vi "TestAxes.vi"(8 "error in (no error)":errorcluster) -> (0 "error out":errorcluster)   [LabVIEW 2009]
uses:
  typedefs/Position3d.ctl
  typedefs/AxesTestSettings.ctl
  typedefs/Ultra3000/Fault_Cluster.ctl
  typedefs/Ultra3000/RunStatus_Ring.ctl
  typedefs/Ultra3000/IndexType.ctl
  typedefs/Ultra3000/HostControlModeRing.ctl
  typedefs/AxisSelect_Enum.ctl
  typedefs/Ultra3000/Index_Numeric.ctl
  typedefs/Ultra3000/IndexTermination.ctl
  typedefs/Ultra3000/AdditionalIndexSettings_Cluster.ctl
panel:
  in  "Y Enable toggle":bool
  in  "Z Enable Toggle":bool
  in  "X Enable toggle":bool
  in  "Axis Settings":T1=[{"Velocity"=5.0, "Accel. / Decel."=5.0, "Dwell"=0}, {"Velocity"=5.0, "Accel. / Decel."=5.0, "Dwell"=0}, {"Velocity"=5.0, "Accel. / Decel."=5.0, "Dwell"=0}]
  in  "Index Type (Absolute)":T2=1 items=["Incremental", "Absolute"]
  in  "Home":bool
  in  "Position 2 (mm)":T3
  in  "Position 1 (mm)":T3
  out "Current (X,Y,Z) Position":string
  in  "stop":bool
  in  "cycle":bool caption="(Hold to start)"
  in  "Move to pos2":bool
  in  "Move to pos1":bool
  in  "Clear Faults":bool
  out "Run Status":T4[](array[typedef]) {"Run Status Description" items=["Fault detected"=1, "Disabled and not faulted"=255, "Enabled"=0]}
  in  "Done":bool
  # "X-Axis Settings"
  # "Y-Axis Settings"
  # "Z-Axis Settings"
  # "X-Axis Run Status"
  # "Y-Axis Run Status"
  # "Z-Axis Run Status"
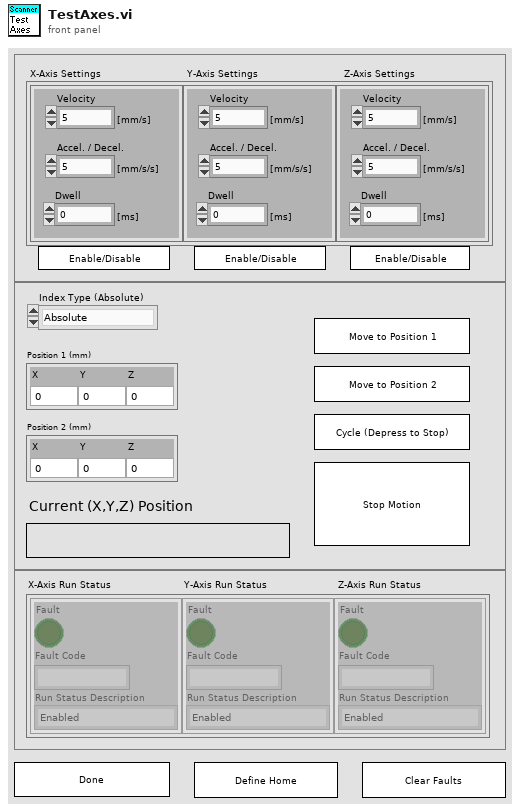
[diagram p1: front panel]
types:
  T1 = typedef "AxesTestSettings.ctl" = cluster{"Velocity":dbl, "Accel. / Decel.":dbl, "Dwell":u16}[]
  T2 = typedef "IndexType.ctl" = i32
  T3 = typedef "Position3d.ctl" = cluster{"X":dbl, "Y":dbl, "Z":dbl}
  T4 = typedef "Fault_Cluster.ctl" = cluster{"Fault":bool, "Fault Code":string, "Run Status Description":T5}
  T5 = typedef "RunStatus_Ring.ctl" = u16
  T6 = typedef "AxisSelect_Enum.ctl" = enum16{"X", "Y", "Z", "Axis Space"}
  T7 = typedef "HostControlModeRing.ctl" = u16
  T8 = typedef "Index_Numeric.ctl" = u8
  T9 = typedef "DriveStatus_Cluster.ctl" = cluster{"In-position":bool, "Zero Speed":bool, "Enabled":bool, "Fault Disable":bool, "Ready":bool, "Start Index":bool, "Overtravel Exceeded":bool, "Up to Speed":bool, "Sequence Complete":bool}
  T10 = enum8{"Enabled", "Disabled", "Disabled and Grayed Out"}
  T11 = typedef "IndexTermination.ctl" = i32
  T12 = typedef "AdditionalIndexSettings_Cluster.ctl" = cluster{"Next Index":u8, "Termination":T11, "Count":u16}
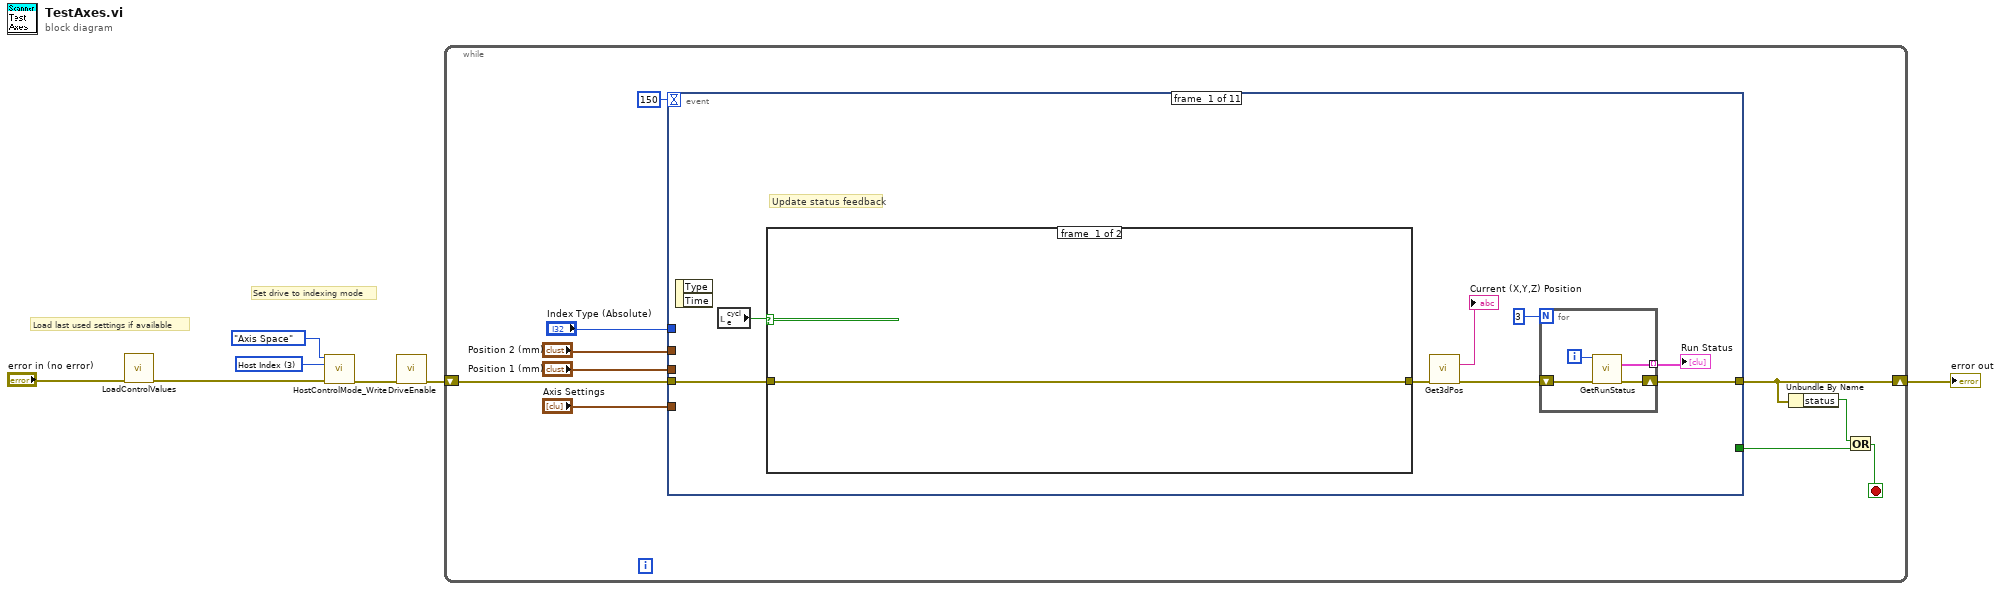
[diagram p0: block diagram]
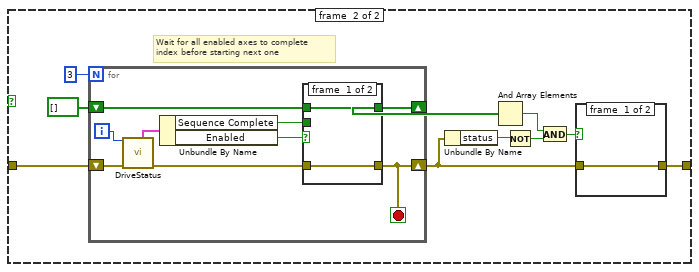
[diagram p2: hidden frame]
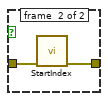
[diagram p3: hidden frame]
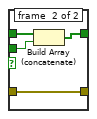
[diagram p4: hidden frame]
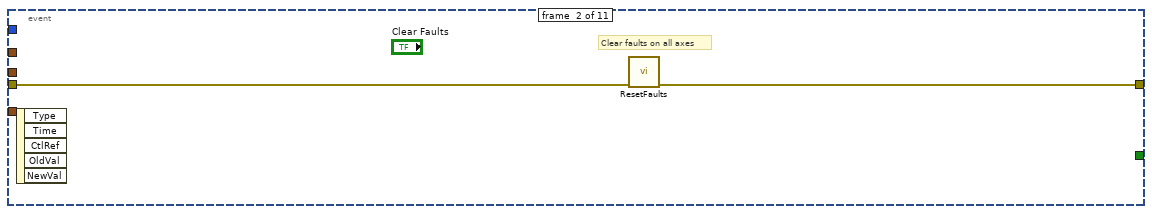
[diagram p5: hidden frame]
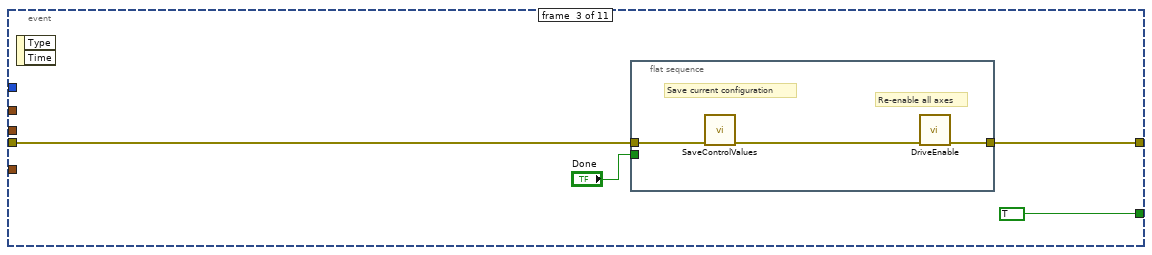
[diagram p6: hidden frame]
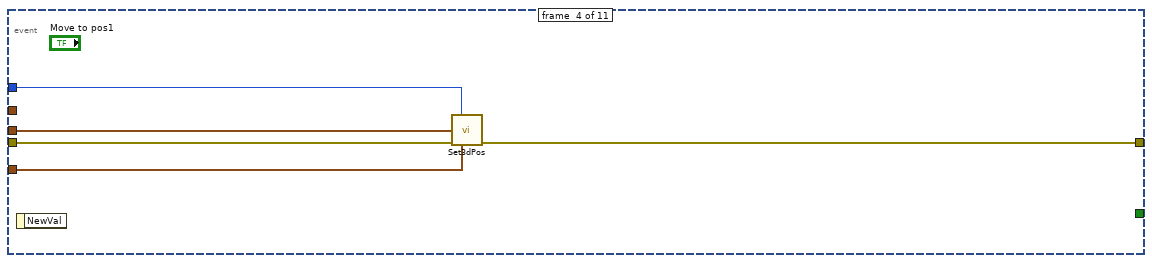
[diagram p7: hidden frame]
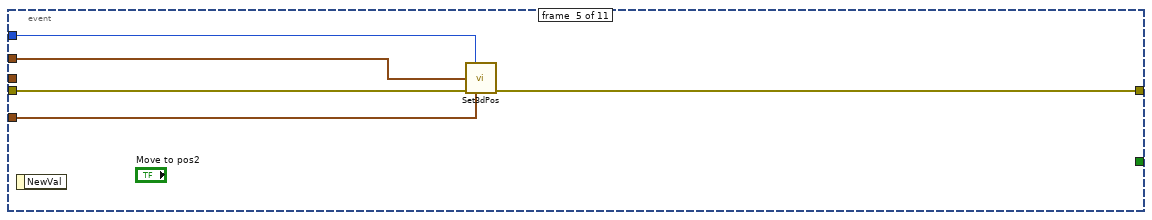
[diagram p8: hidden frame]
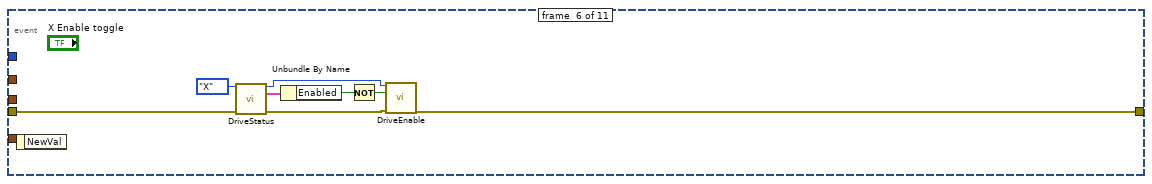
[diagram p9: hidden frame]
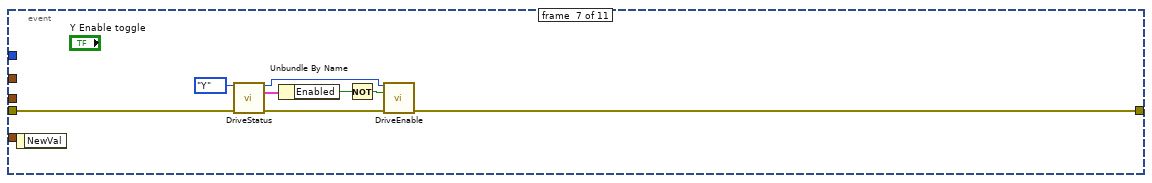
[diagram p10: hidden frame]
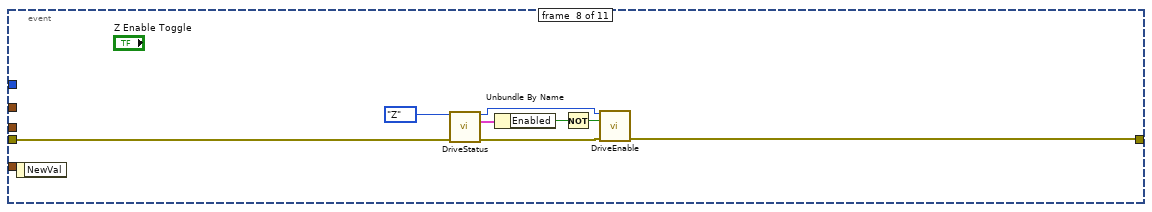
[diagram p11: hidden frame]
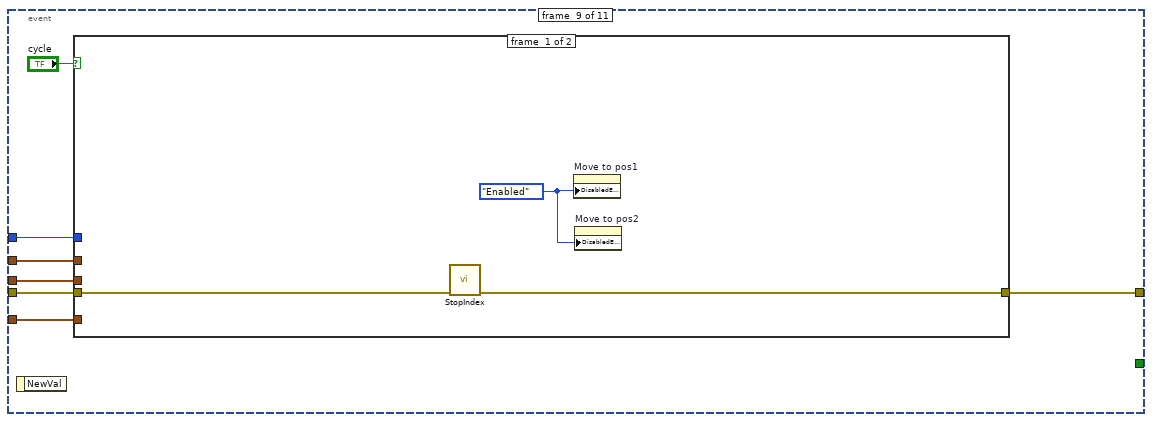
[diagram p12: hidden frame]
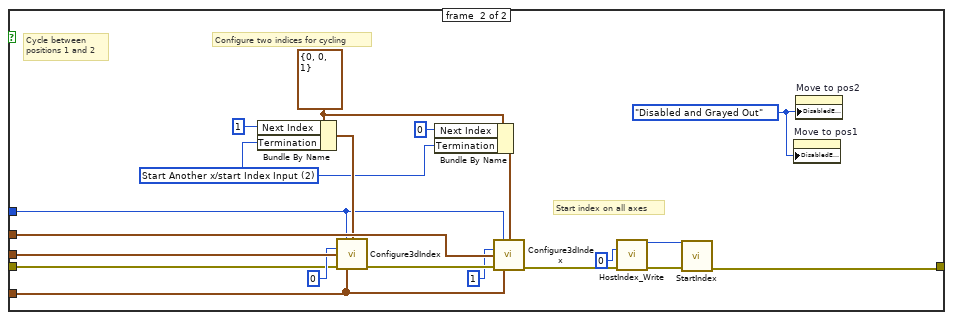
[diagram p13: hidden frame]
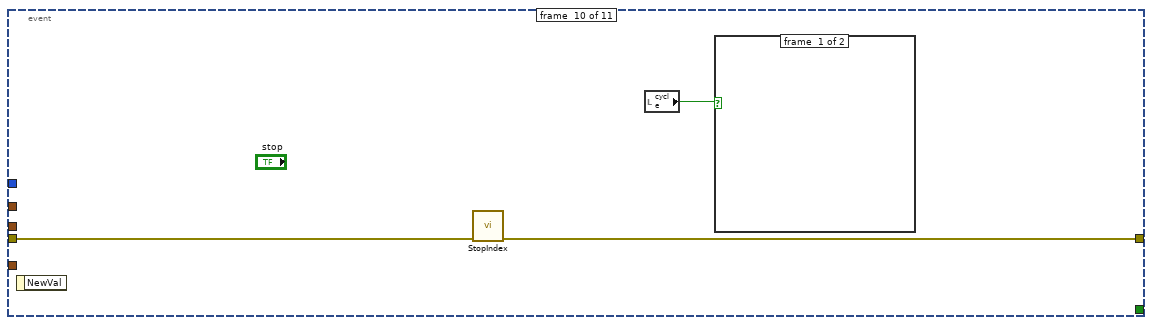
[diagram p14: hidden frame]
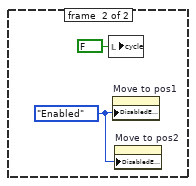
[diagram p15: hidden frame]
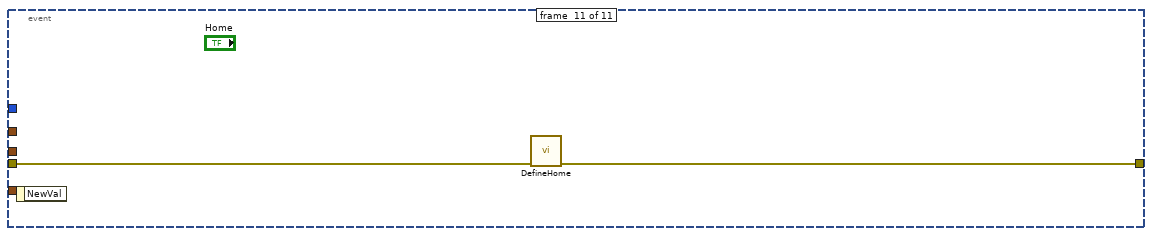
[diagram p16: hidden frame]
diagram:
  w6 = T7 3 items=["Normal Mode", "Setpoint velocity", "Setpoint current", "Host Index"] ("Host Control Mode (Normal)")
  # "Set drive to indexing mode"
  # "Load last used settings if available"
  n1 = call "LoadControlValues.vi"("error in (no error)"="error in (no error)") -> ("error out"=w2:errorcluster)  [unwired: 9 in, 1 out]
  n2 = call "HostControlMode_Write.vi"("Axis In"=AxisSelect_Enum."Axis Space", "Host Control Mode (Normal)"=w6, "error in (no error)"=w2) -> ("error out"=w5:errorcluster)  [unwired: 11 in, 1 out]
  n3 = call "DriveEnable.vi"("error in (no error)"=w5) -> ("error out"=w1:errorcluster)  [unwired: 13 in, 1 out]
  n4 = while {
    shift-right: [w10] -> w4
    shift-left: w1 -> [w11]
    stop <- w12 stop-if-true
    n5 = event shown="[2] \"Done\": Value Change;  Panel Close" {
      selector: _ -> [_ _ _ _ _ _ _ _ _ _ _]
      dyn-events: _ -> [_ _ _ _ _ _ _ _ _ _ _]
      timeout: 150 -> [_ _ _ _ _ _ _ _ _ _ _]
      tunnel: "Axis Settings" -> [_ _ _ w72 w77 _ _ _ w107 _ _]
      tunnel: "Index Type (Absolute)" -> [_ _ _ w71 w76 _ _ _ w106 _ _]
      tunnel: "Position 1 (mm)" -> [_ _ _ w70 _ _ _ _ w108 _ _]
      tunnel: "Position 2 (mm)" -> [_ _ _ _ w75 _ _ _ w105 _ _]
      tunnel: [_ _ TRUE ("x") _ _ _ _ _ _ _ _] -> w8
      tunnel: [w20 w60 w61 w69 w74 w79 w87 w95 w103 w134 w138] -> w10
      tunnel: w11 -> [w18 w59 w62 w68 w73 w78 w86 w94 w102 w132 w137]
      event #0 {
        # "Update status feedback"
        n6 = event-data() -> ()  [unwired: 1 in, 2 out]
        n7 = local read "cycle"() -> (w22:bool)
        n8 = case shown="True" w22 {
          tunnel: [w26 w33] -> w21
          tunnel: w18 -> [w26 w27]
          frame #0 {
          }
          frame #1 {
            # "Wait for all enabled axes to complete\nindex before starting next one"
            n9 = for {
              N: 3 -> [_]
              shift-right: [w48] -> w34
              shift-left: bool[] [] -> [w47]
              shift-right: [w40] -> w28
              shift-left: w27 -> [w41]
              i -> [w45]
              stop <- w40 stop-if-true
              n10 = call "DriveStatus.vi"("Axis In"=w45, "error in (no error)"=w41) -> ("Status"=w46:T9, "error out"=w44:errorcluster)  [unwired: 11 in, 1 out]
              n11 = Unbundle By Name(w46) -> ("Sequence Complete"=w42:bool, "Enabled"=w43:bool)
              n12 = case shown="True" w43 {
                tunnel: [w50 w54] -> w48
                tunnel: w47 -> [w50 w53]
                tunnel: w44 -> [w49 w51]
                tunnel: [w49 w51] -> w40
                tunnel: w42 -> [_ w52]
                frame #0 {
                }
                frame #1 {
                  n13 = Build Array (concatenate)(w53, w52) -> (w54:bool[])
                }
              }
            }
            n14 = Unbundle By Name(w28) -> ("status"=w29:bool)
            n15 = And Array Elements(Boolean array=w34) -> (logical AND=w32:bool)
            n16 = Not(x=w29) -> (.not. x?=w30:bool)
            n17 = And(x=w32, y=w30) -> (x .and. y?=w31:bool)
            n18 = case shown="True" w31 {
              tunnel: [w37 w39] -> w33
              tunnel: w28 -> [w37 w38]
              frame #0 {
              }
              frame #1 {
                n19 = call "StartIndex.vi"("error in (no error)"=w38) -> ("error out"=w39:errorcluster)  [unwired: 13 in, 1 out]
              }
            }
          }
        }
        n20 = call "Get3dPos.vi"("error in (no error)"=w21) -> ("(X,Y,Z) Position"=→"Current (X,Y,Z) Position":string, "error out"=w24:errorcluster)  [unwired: 13 in]
        n21 = for {
          N: 3 -> [_]
          shift-right: [w56] -> w20
          shift-left: w24 -> [w57]
          tunnel: [w55] -> w19 mode=indexing
          i -> [w58]
          n22 = call "GetRunStatus.vi"("Axis In"=w58, "error in (no error)"=w57) -> ("run status"=w55:T4, "error out"=w56:errorcluster)  [unwired: 11 in, 1 out]
        }
        "Run Status" <- w19
      }
      event #1 {
        # "Clear faults on all axes"
        n23 = event-data() -> ()  [unwired: 1 in, 5 out]
        n24 = call "ResetFaults.vi"("error in (no error)"=w59) -> ("error out"=w60:errorcluster)  [unwired: 13 in, 1 out]
      }
      event #2 {
        n25 = event-data() -> ()  [unwired: 1 in, 2 out]
        n26 = flat-sequence {
          tunnel: "Done" -> [_]
          tunnel: w62 -> [w67]
          tunnel: [w65] -> w61
          frame #0 {
            # "Re-enable all axes"
            # "Save current configuration"
            n27 = call "SaveControlValues.vi"("error in"=w67) -> ("error out"=w66:errorcluster)  [unwired: 8 in]
            n28 = call "DriveEnable.vi"("error in (no error)"=w66) -> ("error out"=w65:errorcluster)  [unwired: 13 in, 1 out]
          }
        }
      }
      event #3 {
        n29 = event-data() -> ()  [unwired: 1 in, 1 out]
        n30 = call "Set3dPos.vi"("Index Type (Absolute)"=w71, "Position (mm)"=w70, "error in (no error)"=w68, "Axis Settings"=w72) -> ("error out"=w69:errorcluster)  [unwired: 10 in, 1 out]
      }
      event #4 {
        n31 = event-data() -> ()  [unwired: 1 in, 1 out]
        n32 = call "Set3dPos.vi"("Index Type (Absolute)"=w76, "Position (mm)"=w75, "error in (no error)"=w73, "Axis Settings"=w77) -> ("error out"=w74:errorcluster)  [unwired: 10 in, 1 out]
      }
      event #5 {
        n33 = event-data() -> ()  [unwired: 1 in, 1 out]
        n34 = call "DriveStatus.vi"("Axis In"=AxisSelect_Enum."X" ("Axis In (Axis Space)"), "error in (no error)"=w78) -> ("Axis Out"=w83:T6, "Status"=w82:T9, "error out"=w84:errorcluster)  [unwired: 11 in]
        n35 = Unbundle By Name(w82) -> ("Enabled"=w81:bool)
        n36 = Not(x=w81) -> (.not. x?=w80:bool)
        n37 = call "DriveEnable.vi"("Axis In (Axis Space)"=w83, "Enable (T)"=w80, "error in (no error)"=w84) -> ("error out"=w79:errorcluster)  [unwired: 11 in, 1 out]
      }
      event #6 {
        n38 = event-data() -> ()  [unwired: 1 in, 1 out]
        n39 = call "DriveStatus.vi"("Axis In"=AxisSelect_Enum."Y" ("Axis In (Axis Space)"), "error in (no error)"=w86) -> ("Axis Out"=w91:T6, "Status"=w90:T9, "error out"=w92:errorcluster)  [unwired: 11 in]
        n40 = Unbundle By Name(w90) -> ("Enabled"=w89:bool)
        n41 = Not(x=w89) -> (.not. x?=w88:bool)
        n42 = call "DriveEnable.vi"("Axis In (Axis Space)"=w91, "Enable (T)"=w88, "error in (no error)"=w92) -> ("error out"=w87:errorcluster)  [unwired: 11 in, 1 out]
      }
      event #7 {
        n43 = event-data() -> ()  [unwired: 1 in, 1 out]
        n44 = call "DriveStatus.vi"("Axis In"=AxisSelect_Enum."Z" ("Axis In (Axis Space)"), "error in (no error)"=w94) -> ("Axis Out"=w99:T6, "Status"=w98:T9, "error out"=w100:errorcluster)  [unwired: 11 in]
        n45 = Unbundle By Name(w98) -> ("Enabled"=w97:bool)
        n46 = Not(x=w97) -> (.not. x?=w96:bool)
        n47 = call "DriveEnable.vi"("Axis In (Axis Space)"=w99, "Enable (T)"=w96, "error in (no error)"=w100) -> ("error out"=w95:errorcluster)  [unwired: 11 in, 1 out]
      }
      event #8 {
        n48 = event-data() -> ()  [unwired: 1 in, 1 out]
        n49 = case shown="True" "cycle" {
          tunnel: w108 -> [_ w131]
          tunnel: w107 -> [_ w130]
          tunnel: w106 -> [_ w112]
          tunnel: w105 -> [_ w129]
          tunnel: [w110 w114] -> w103
          tunnel: w102 -> [w109 w113]
          frame #0 {
            w111 = T10."Enabled" ("Disabled")
            n50 = call "StopIndex.vi"("error in (no error)"=w109) -> ("error out"=w110:errorcluster)  [unwired: 13 in, 1 out]
            n51 = property on="Move to pos1" class="Bool"("DisabledEnum"=w111) -> ()  [unwired: 2 in, 2 out]
            n52 = property on="Move to pos2" class="Bool"("DisabledEnum"=w111) -> ()  [unwired: 2 in, 2 out]
          }
          frame #1 {
            w124 = T10."Disabled and Grayed Out" ("Disabled")
            w119 = T11 2 items=["Stop", "Start Another Immediately", "Start Another x/start Index Input", "Start Another Index Without Stopping"] ("Termination")
            w122 = T12 {"Next Index"=0, "Termination"=0, "Count"=1} ("Additional Settings")
            # "Start index on all axes"
            # "Configure two indices for cycling"
            # "Cycle between\npositions 1 and 2"
            n53 = Bundle By Name(cluster=w122, "Next Index"=u8 1, "Termination"=w119) -> (w127:T12)
            n54 = call "Configure3dIndex.vi"("Index Type (Absolute)"=w112, "Additional Settings"=w127, "Index (0)"=T8 0 ("Index"), "Position"=w131, "error in (no error)"=w113, "Axis Settings"=w130) -> ("error out"=w128:errorcluster)  [unwired: 8 in, 1 out]
            n55 = Bundle By Name(cluster=w122, "Next Index"=u8 0, "Termination"=w119) -> (w123:T12)
            n56 = call "Configure3dIndex.vi"("Index Type (Absolute)"=w112, "Additional Settings"=w123, "Index (0)"=T8 1 ("Index"), "Position"=w129, "error in (no error)"=w128, "Axis Settings"=w130) -> ("error out"=w125:errorcluster)  [unwired: 8 in, 1 out]
            n57 = call "HostIndex_Write.vi"("Index"=T8 0, "error in (no error)"=w125) -> ("Axis Out"=w115:T6, "error out"=w116:errorcluster)  [unwired: 11 in, 1 out]
            n58 = call "StartIndex.vi"("Axis In (Axis Space)"=w115, "error in (no error)"=w116) -> ("error out"=w114:errorcluster)  [unwired: 12 in, 1 out]
            n59 = property on="Move to pos1" class="Bool"("DisabledEnum"=w124) -> ()  [unwired: 2 in, 2 out]
            n60 = property on="Move to pos2" class="Bool"("DisabledEnum"=w124) -> ()  [unwired: 2 in, 2 out]
          }
        }
      }
      event #9 {
        n61 = event-data() -> ()  [unwired: 1 in, 1 out]
        n62 = call "StopIndex.vi"("error in (no error)"=w132) -> ("error out"=w134:errorcluster)  [unwired: 13 in, 1 out]
        n63 = local read "cycle"() -> (w133:bool)
        n64 = case shown="True" w133 {
          frame #0 {
          }
          frame #1 {
            w135 = T10."Enabled" ("Disabled")
            n65 = local write "cycle"(FALSE ("cycle")) -> ()
            n66 = property on="Move to pos1" class="Bool"("DisabledEnum"=w135) -> ()  [unwired: 2 in, 2 out]
            n67 = property on="Move to pos2" class="Bool"("DisabledEnum"=w135) -> ()  [unwired: 2 in, 2 out]
          }
        }
      }
      event #10 {
        n68 = event-data() -> ()  [unwired: 1 in, 1 out]
        n69 = call "DefineHome.vi"("error in (no error)"=w137) -> ("error out"=w138:errorcluster)  [unwired: 13 in, 1 out]
      }
    }
    n70 = Unbundle By Name(w10) -> ("status"=w9:bool)
    n71 = Or(x=w9, y=w8) -> (x .or. y?=w12:bool)
  }
  "error out" <- w4
